vi "Parse DB - 1553 - Get BC Config.vi"(0 "channel config handle":u32, 11 "error in (no error)":errorcluster) -> (4 "channel config handle out":u32, 6 "Bus_Controller":T1, 8 "Xfer Count != Buffer Count":bool, 15 "error out":errorcluster)   [LabVIEW 2013]
uses:
  Controls/1553_Bus_Controller.ctl
  Controls/1553_BC_Message.ctl
  Controls/664 -Param.ctl
  Controls/1553_Acyclic_Frame.ctl
  <userlib>/MIL-STD-1553/Owl1553.lvlib
  AIT 664 Custom Device.lvlib
panel:
  out "description":string
  out "Xfer count":u32
  out "buffer count":u32
  out "BC Initial Buffer Data":u16[][](array[numeric]) format="%.0x"
  out "BC Sizes":u32[](array[numeric])
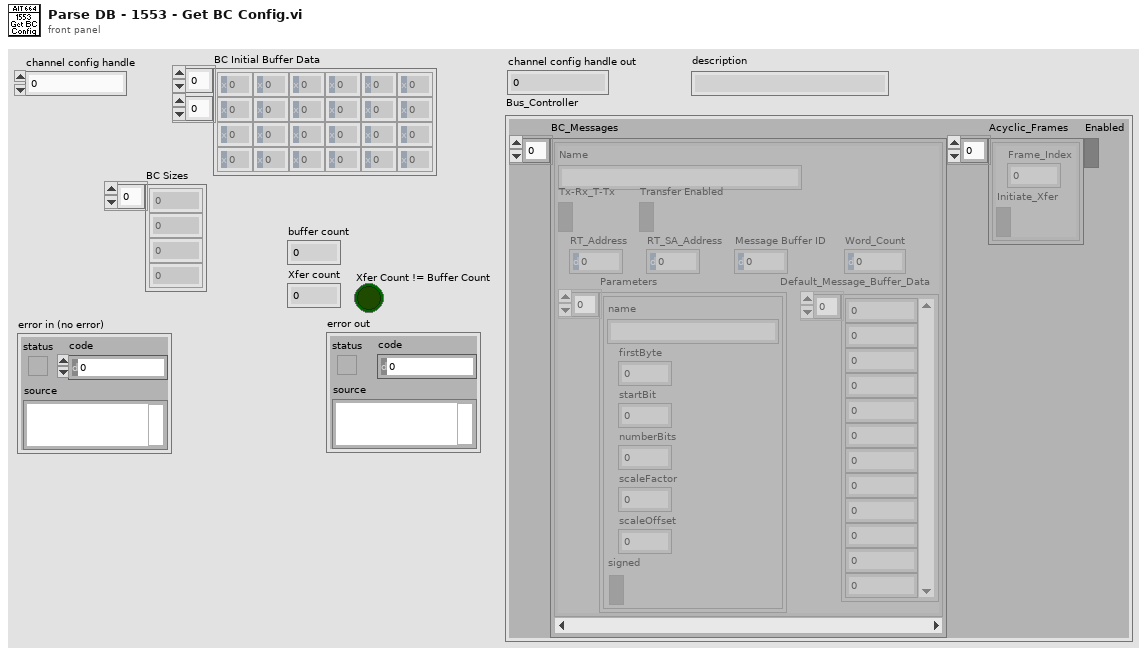
[diagram p1: front panel]
types:
  T1 = typedef "AIT 664 Custom Device.lvlib/1553_Bus_Controller.ctl" = cluster{"BC_Messages":T2[], "Acyclic_Frames":T4[], "Enabled":bool}
  T2 = typedef "AIT 664 Custom Device.lvlib/1553_BC_Message.ctl" = cluster{"Name":string, "Tx-Rx_T-Tx":bool, "RT_Address":u8, "RT_SA_Address":u8, "Parameters":T3[], "Transfer Enabled":bool, "Message Buffer ID":u16, "Default_Message_Buffer_Data":u16[], "Word_Count":u8}
  T3 = typedef "AIT 664 Custom Device.lvlib/664 -Param.ctl" = cluster{"name":string, "firstByte":i32, "startBit":i32, "numberBits":i32, "scaleFactor":dbl, "scaleOffset":dbl, "signed":bool}
  T4 = typedef "AIT 664 Custom Device.lvlib/1553_Acyclic_Frame.ctl" = cluster{"Frame_Index":u8, "Initiate_Xfer":bool}
  T5 = enum16{"OWL1553_BCRT", "OWL1553_RTBC", "OWL1553_RTRT", "OWL1553_FRONT_HALF", "OWL1553_BACK_HALF", "OWL1553_MSG_ERROR"}
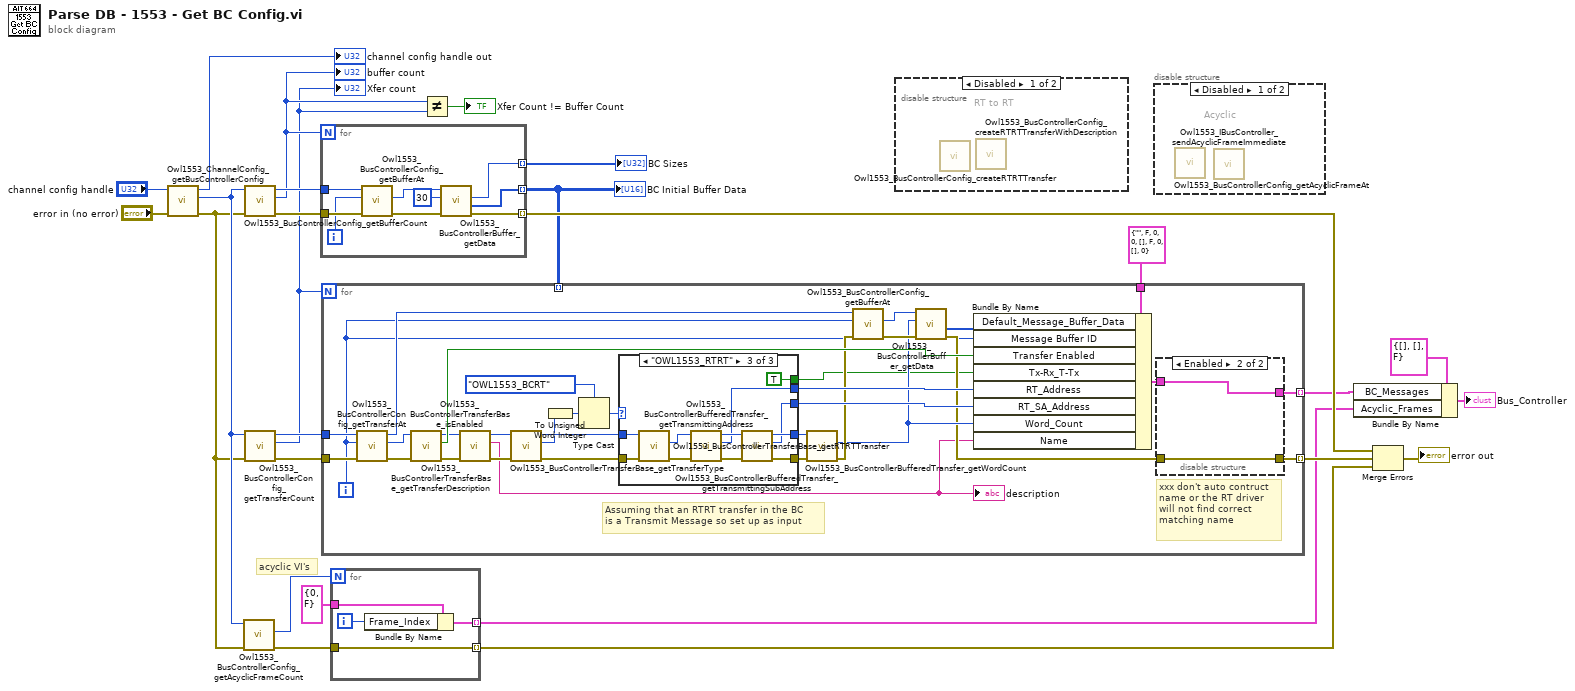
[diagram p0: block diagram]
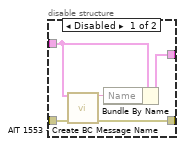
[diagram p4: hidden frame]
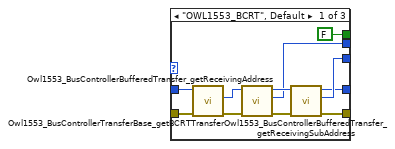
[diagram p5: hidden frame]
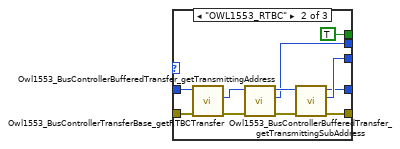
[diagram p6: hidden frame]
diagram:
  # "acyclic VI's"
  n1 = call <userlib>:"Owl1553_ChannelConfig_getBusControllerConfig.vi"("error in (no error)"="error in (no error)", "channel config handle"="channel config handle") -> ("error out"=w6:errorcluster, "bus controller config handle"=w7:u64, "channel config handle"=→"channel config handle out":u64)  [unwired: 7 in]
  n2 = call <userlib>:"Owl1553_BusControllerConfig_getAcyclicFrameCount.vi"("error in (no error)"=w6, "bus controller config handle"=w7) -> ("error out"=w4:errorcluster, "acyclic frame count"=w5:u32)  [unwired: 7 in, 1 out]
  n3 = call <userlib>:"Owl1553_BusControllerConfig_getBufferCount.vi"("error in (no error)"=w6, "bus controller config handle"=w7) -> ("error out"=w25:errorcluster, "buffer count"=w18:u32, "bus controller config handle"=w24:u64)  [unwired: 7 in]
  "buffer count" <- w18
  n4 = call <userlib>:"Owl1553_BusControllerConfig_getTransferCount.vi"("error in (no error)"=w6, "bus controller config handle"=w7) -> ("error out"=w21:errorcluster, "transfer count"=w9:u32, "bus controller config handle"=w20:u64)  [unwired: 7 in]
  "Xfer count" <- w9
  n5 = for {
    N: w18 -> [_]
    tunnel: w24 -> [w35]
    tunnel: w25 -> [w34]
    tunnel: [w27] -> w14 mode=indexing
    tunnel: [w32] -> w26 mode=indexing
    tunnel: [w31] -> w15 mode=indexing
    i -> [w33]
    n6 = call <userlib>:"Owl1553_BusControllerConfig_getBufferAt.vi"("error in (no error)"=w34, "index"=w33, "bus controller config handle"=w35) -> ("error out"=w30:errorcluster, "buffer handle"=w29:u64)  [unwired: 6 in, 1 out]
    n7 = call <userlib>:"Owl1553_BusControllerBuffer_getData.vi"("error in (no error)"=w30, "buffer size"=u32 30, "bus controller buffer handle"=w29) -> ("error out"=w31:errorcluster, "data"=w27:u16[], "buffer size out"=w32:u32)  [unwired: 5 in, 1 out]
  }
  "BC Initial Buffer Data" <- w14
  "BC Sizes" <- w26
  n8 = for {
    N: w9 -> [_]
    tunnel: w20 -> [w63]
    tunnel: w21 -> [w68]
    tunnel: T2 {"Name"="", "Tx-Rx_T-Tx"=FALSE, "RT_Address"=0, "RT_SA_Address"=0, "Parameters"=[], "Transfer Enabled"=FALSE, "Message Buffer ID"=0, "Default_Message_Buffer_Data"=[], "Word_Count"=0} ("BC_Message") -> [w60]
    tunnel: [w56] -> w16 mode=indexing
    tunnel: [w50] -> w12 mode=indexing
    tunnel: w14 -> [_] mode=indexing
    i -> [w42]
    # "Assuming that an RTRT transfer in the BC\nis a Transmit Message so set up as input"
    # "xxx don't auto contruct\nname or the RT driver\nwill not find correct\nmatching name"
    n9 = call <userlib>:"Owl1553_BusControllerConfig_getTransferAt.vi"("error in (no error)"=w68, "index"=w42, "bus controller config handle"=w63) -> ("error out"=w64:errorcluster, "transfer base handle"=w61:u64, "bus controller config handle"=w43:u64)  [unwired: 6 in]
    n10 = call <userlib>:"Owl1553_BusControllerTransferBase_isEnabled.vi"("error in (no error)"=w64, "transferbase handle"=w61) -> ("error out"=w53:errorcluster, "enabled"=w55:bool, "transferbase handle"=w54:u64)  [unwired: 6 in]
    n11 = call "Owl1553_BusControllerTransferBase_getTransferDescription.vi"("error in (no error)"=w53, "transferbase handle"=w54) -> ("error out"=w52:errorcluster, "transferdescription"=w40:string, "transferbase handle"=w51:u32)  [unwired: 6 in]
    "description" <- w40
    n12 = call <userlib>:"Owl1553_BusControllerTransferBase_getTransferType.vi"("error in (no error)"=w52, "transferbase handle"=w51) -> ("error out"=w66:errorcluster, "transfer type"=w38:i32, "transferbase handle"=w62:u64)  [unwired: 6 in]
    n13 = To Unsigned Word Integer(number=w38) -> (unsigned 16bit integer=w41:u16)
    n14 = Type Cast(type=T5."OWL1553_BCRT" ("Owl1553TransferMessageType"), x=w41) -> (*(type *) &x=w37:T5)
    n15 = case shown="\"OWL1553_RTRT\"" w37 {
      tunnel: w66 -> [w86 w97 w107]
      tunnel: [w80 w91 w100] -> w67
      tunnel: [w79 w92 w99] -> w65
      tunnel: w62 -> [w85 w96 w108]
      tunnel: [w82 w90 w102] -> w58
      tunnel: [w81 w93 w98] -> w59
      tunnel: [FALSE ("Initiate_Xfer") TRUE ("Initiate_Xfer") TRUE ("Initiate_Xfer")] -> w36
      frame "OWL1553_BCRT", Default {
        n16 = call <userlib>:"Owl1553_BusControllerTransferBase_getBCRTTransfer.vi"("error in (no error)"=w86, "transferbase handle"=w85) -> ("error out"=w78:errorcluster, "bcrt transfer handle"=w77:u64)  [unwired: 6 in, 1 out]
        n17 = call <userlib>:"Owl1553_BusControllerBufferedTransfer_getReceivingAddress.vi"("error in (no error)"=w78, "buffered transfer handle"=w77) -> ("error out"=w84:errorcluster, "remote terminal address"=w82:u8, "buffered transfer handle"=w83:u64)  [unwired: 6 in]
        n18 = call <userlib>:"Owl1553_BusControllerBufferedTransfer_getReceivingSubAddress.vi"("error in (no error)"=w84, "buffered transfer handle"=w83) -> ("error out"=w80:errorcluster, "remote terminal address"=w81:u8, "buffered transfer handle"=w79:u64)  [unwired: 6 in]
      }
      frame "OWL1553_RTBC" {
        n19 = call <userlib>:"Owl1553_BusControllerTransferBase_getRTBCTransfer.vi"("error in (no error)"=w97, "transferbase handle"=w96) -> ("error out"=w88:errorcluster, "rtbc transfer handle"=w89:u64)  [unwired: 6 in, 1 out]
        n20 = call <userlib>:"Owl1553_BusControllerBufferedTransfer_getTransmittingAddress.vi"("error in (no error)"=w88, "buffered transfer handle"=w89) -> ("error out"=w95:errorcluster, "remote terminal address"=w90:u8, "buffered transfer handle"=w94:u64)  [unwired: 6 in]
        n21 = call <userlib>:"Owl1553_BusControllerBufferedTransfer_getTransmittingSubAddress.vi"("error in (no error)"=w95, "buffered transfer handle"=w94) -> ("error out"=w91:errorcluster, "remote terminal sub-address"=w93:u8, "buffered transfer handle"=w92:u64)  [unwired: 6 in]
      }
      frame "OWL1553_RTRT" {
        n22 = call <userlib>:"Owl1553_BusControllerTransferBase_getRTRTTransfer.vi"("error in (no error)"=w107, "transferbase handle"=w108) -> ("error out"=w103:errorcluster, "rtrt transfer handle"=w104:u64)  [unwired: 6 in, 1 out]
        n23 = call <userlib>:"Owl1553_BusControllerBufferedTransfer_getTransmittingAddress.vi"("error in (no error)"=w103, "buffered transfer handle"=w104) -> ("error out"=w101:errorcluster, "remote terminal address"=w102:u8, "buffered transfer handle"=w105:u64)  [unwired: 6 in]
        n24 = call <userlib>:"Owl1553_BusControllerBufferedTransfer_getTransmittingSubAddress.vi"("error in (no error)"=w101, "buffered transfer handle"=w105) -> ("error out"=w100:errorcluster, "remote terminal sub-address"=w98:u8, "buffered transfer handle"=w99:u64)  [unwired: 6 in]
      }
    }
    n25 = call <userlib>:"Owl1553_BusControllerBufferedTransfer_getWordCount.vi"("error in (no error)"=w67, "buffered transfer handle"=w65) -> ("error out"=w47:errorcluster, "word count"=w46:u8)  [unwired: 6 in, 1 out]
    n26 = call <userlib>:"Owl1553_BusControllerConfig_getBufferAt.vi"("error in (no error)"=w47, "index"=w42, "bus controller config handle"=w43) -> ("error out"=w48:errorcluster, "buffer handle"=w49:u64)  [unwired: 6 in, 1 out]
    n27 = call <userlib>:"Owl1553_BusControllerBuffer_getData.vi"("error in (no error)"=w48, "buffer size"=w46, "bus controller buffer handle"=w49) -> ("error out"=w44:errorcluster, "data"=w45:u16[])  [unwired: 5 in, 2 out]
    n28 = Bundle By Name(cluster=w60, "Default_Message_Buffer_Data"=w45, "Message Buffer ID"=w42, "Transfer Enabled"=w55, "Tx-Rx_T-Tx"=w36, "RT_Address"=w58, "RT_SA_Address"=w59, "Word_Count"=w46, "Name"=w40) -> (w57:T2)
    n29 = disable-structure shown="Enabled" {
      disable-tunnel: w57 -> [w73 w75]
      disable-tunnel: w44 -> [w72 w74]
      disable-tunnel: [w71 w74] -> w56
      disable-tunnel: [w69 w75] -> w50
      frame Disabled {
        n30 = call "AIT 1553 - Create BC Message Name.vi"("BC_Message"=w73, "error in (no error)"=w72) -> ("Message Name"=w70:string, "error out"=w71:errorcluster)  [unwired: 12 in]
        n31 = Bundle By Name(cluster=w73, "Name"=w70) -> (w69:T2)
      }
      frame Enabled {
      }
    }
  }
  n32 = for {
    N: w5 -> [_]
    tunnel: w4 -> [w110]
    tunnel: T4 {"Frame_Index"=0, "Initiate_Xfer"=FALSE} ("Acyclic_Frame") -> [w112]
    tunnel: [w110] -> w2 mode=indexing
    tunnel: [w109] -> w1 mode=indexing
    i -> [w111]
    n33 = Bundle By Name(cluster=w112, "Frame_Index"=w111) -> (w109:T4)
  }
  n34 = Not Equal?(x=w18, y=w9) -> (x != y?=→"Xfer Count != Buffer Count":bool)
  n35 = disable-structure shown="Disabled" {
    frame Disabled {
      # "RT to RT"
      n36 = call <userlib>:"Owl1553_BusControllerConfig_createRTRTTransfer.vi"() -> ()  [unwired: 8 in, 4 out]
      n37 = call <userlib>:"Owl1553_BusControllerConfig_createRTRTTransferWithDescription.vi"() -> ()  [unwired: 11 in, 5 out]
    }
    frame Enabled {
    }
  }
  n38 = disable-structure shown="Disabled" {
    frame Disabled {
      # "Acyclic"
      n39 = call <userlib>:"Owl1553_BusControllerConfig_getAcyclicFrameAt.vi"() -> ()  [unwired: 9 in, 3 out]
      n40 = call <userlib>:"Owl1553_IBusController_sendAcyclicFrameImmediate.vi"() -> ()  [unwired: 10 in, 2 out]
    }
    frame Enabled {
    }
  }
  n41 = Bundle By Name(cluster=T1 {"BC_Messages"=[], "Acyclic_Frames"=[], "Enabled"=FALSE} ("Bus_Controller"), "BC_Messages"=w12, "Acyclic_Frames"=w1) -> (→"Bus_Controller":T1)
  n42 = Merge Errors(w15, w16, w2) -> (→"error out":errorcluster)
